vi "Framework Plugin Runtime Test.vi"() -> ()   [LabVIEW 2016]
uses:
  Plugin Runtime.UDP/Plugin Runtime.UDP.lvclass
  Plugin/Plugin.lvclass
  Framework/Framework.lvclass
  <vilib>/platform/TimedLoop/XDataNode/XDataNode.xnode
  <vilib>/Platform/TimedLoop/XDataNode/nitl_modes.ctl
  <vilib>/Platform/TimedLoop/XDataNode/XDNodeRunTimeDep.lvlib
  <vilib>/Platform/TimedLoop/XDataNode/wakeup.ctl
  <vilib>/Platform/TimedLoop/XDataNode/timing_clust.ctl
  Simulated VeriStand Engine/Simulated VeriStand Engine.lvclass
  Typdefs/Decimation Factors.ctl
  <vilib>/NI Veristand/VeriStand Data/Typedefs/Typedefs.Data Types.ctl
  <vilib>/NI Veristand/VeriStand Data/VeriStand Data.lvlib
  <vilib>/NI Veristand/VeriStand Data/Byte Buffer/Byte Buffer.Mapping.ctl
  <vilib>/NI Veristand/VeriStand Data/Byte Buffer/Byte Buffer.lvclass
  Typdefs/Buffer Configuration.ctl
  C:/Git/SourceTree/VeriStand-Data-Sharing-Framework/Prototyping/Plugin Runtime/Plugin Runtime.lvclass
  <vilib>/NI Veristand/Custom Device API/Data Reference.ctl
  <vilib>/NI VeriStand/Custom Device API/Custom Device API.lvlib
panel:
  out "Plugin Base Pointer":u64 format="%016x"
  in  "Engine Loop Rate (Hz)":dbl=100.0 format="%#_13g"
  in  "Engine Channel Count":i64=1000
  in  "Channels per Section":i32=100
  in  "Number of Sections":i32=5
  in  "Plugin Data Offset":T1 format="%.0x"
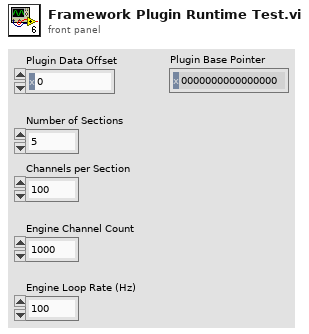
[diagram p1: front panel]
types:
  T1 = typedef "Custom Device API.lvlib/Data Reference.ctl" = i32
  T2 = typedef "Buffer Configuration.ctl" = cluster{"channel mappings":T3[], "rate decimation factors":T5}
  T3 = typedef "VeriStand Data.lvlib/Byte Buffer.lvclass/Byte Buffer.Mapping.ctl" = cluster{"pointer":u64, "count":i64, "buffer offset":u64, "data type":T4}
  T4 = typedef "VeriStand Data.lvlib/Typedefs.Data Types.ctl" = enum16{"Boolean", "Single", "Double", "I8", "I16", "I32", "I64", "U8", "U16", "U32", "U64"}
  T5 = typedef "Decimation Factors.ctl" = cluster{"decimation":u16, "offset":u16}
  T6 = typedef "XDNodeRunTimeDep.lvlib/timing_clust.ctl" = cluster{"Expected End [f-1]":u64, "Actual End [f-1]":u64, "Finished Late? [f-1]":bool, "Expected End [i-1]":u64, "Actual End [i-1]":u64, "Finished Late? [i-1]":bool, "Expected Start [i]":u64, "Actual Start [i]":u64, "Expected Start [f]":u64, "Actual Start [f]":u64, "Source Name":string, "Structure Name":string, "Period":i64, "Deadline":i64, "Offset":i64, "Start":i64, "Priority":i32, "Timeout":i32, "Mode":T7, "Wakeup Reason":T8, "Error":errorcluster, "Source Type":string, "Secondary Source Type":string, "Global End Time":u64, "Global Start Time":u64, "Frame Duration":u64, "Iteration Duration":u64, "Assigned CPU":i32, "I/O Scan Engine Mode":u32}
  T7 = typedef "XDNodeRunTimeDep.lvlib/nitl_modes.ctl" = enum32{"No Change", "Process missed periods, maintain original phase", "Discard missed periods, maintain original phase", "Process missed periods, ignore original phase", "Discard missed periods, ignore original phase"}
  T8 = typedef "XDNodeRunTimeDep.lvlib/wakeup.ctl" = enum32{"Normal", "Aborted", "Asynchronous wakeup", "Timing source error", "Timed loop error", "Timeout"}
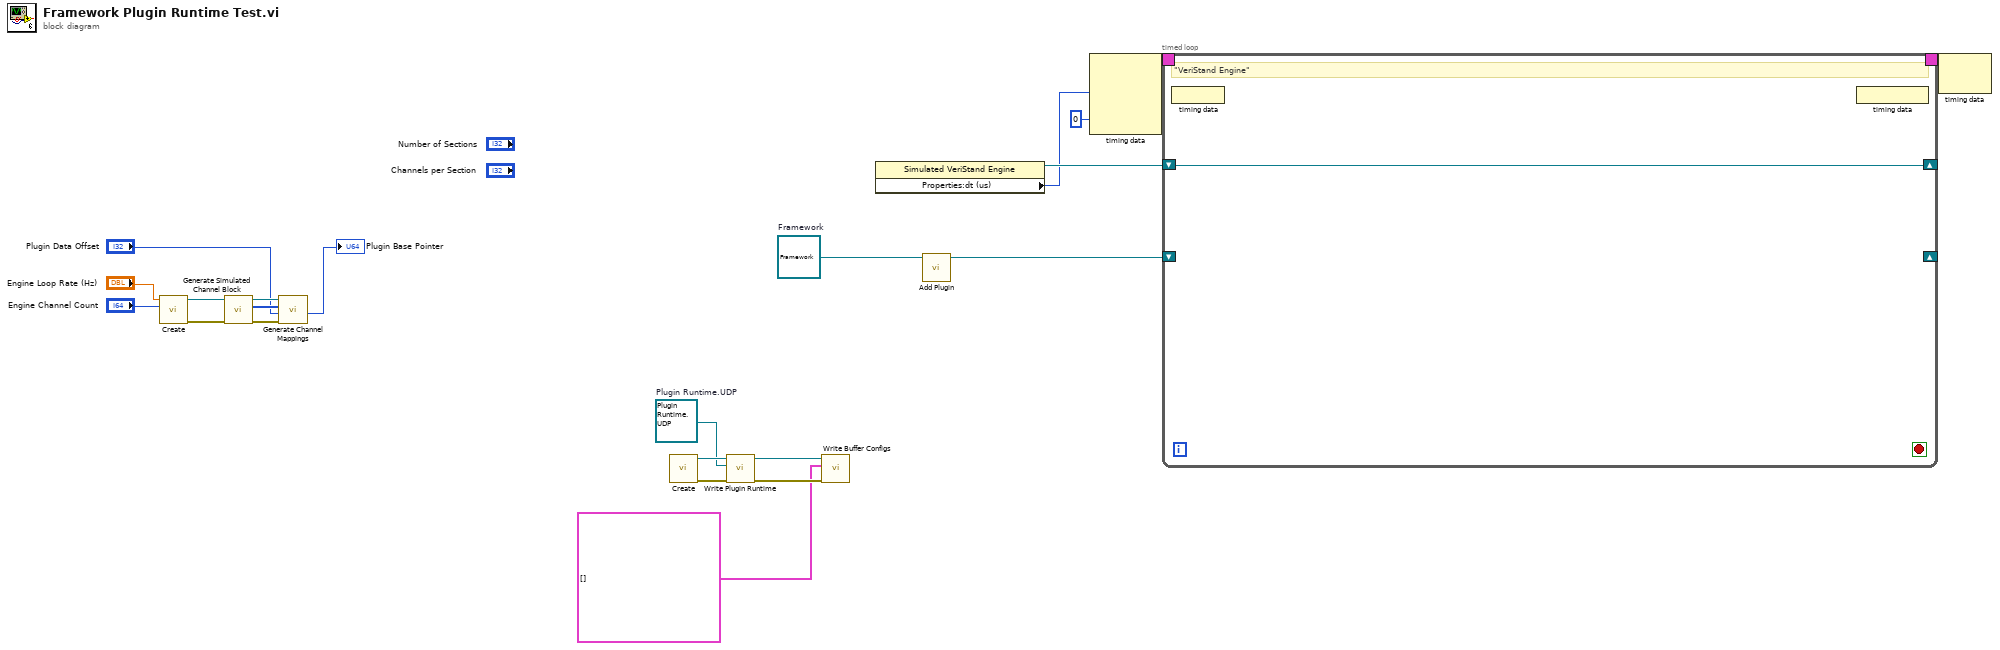
[diagram p0: block diagram]
diagram:
  w12 = refnum<class "Framework.lvclass"> refnum  # Framework
  w13 = refnum<class "Plugin Runtime.UDP.lvclass"> refnum  # Plugin Runtime.UDP
  n1 = call "Create.vi"("Channel Count"="Engine Channel Count", "Loop Rate (Hz)"="Engine Loop Rate (Hz)") -> ("error out"=w6:errorcluster, "Simulated VeriStand Engine out"=w3:refnum<class "Simulated VeriStand Engine.lvclass">)  [unwired: 8 in]
  n2 = call "Generate Simulated Channel Block.vi"("error in (no error)"=w6, "Simulated VeriStand Engine in"=w3) -> ("error out"=w5:errorcluster, "Channels"=w2:T4[], "Simulated VeriStand Engine out"=w4:refnum<class "Simulated VeriStand Engine.lvclass">)  [unwired: 6 in, 1 out]
  n3 = call "Generate Channel Mappings.vi"("error in (no error)"=w5, "Plugin Data Offset"="Plugin Data Offset", "Channels"=w2, "Simulated VeriStand Engine in"=w4) -> ("Base Pointer"=→"Plugin Base Pointer":u64)  [unwired: 4 in, 3 out]
  n4 = call "Create.vi"() -> ("error out"=w14:errorcluster, "Plugin out"=w15:refnum<class "Plugin.lvclass">)  [unwired: 10 in]
  n5 = call "Write Plugin Runtime.vi"("error in (no error)"=w14, "Data Sharing Plugin Runtime"=w13, "Data Sharing Plugin in"=w15) -> ("error out"=w9:errorcluster, "Data Sharing Plugin out"=w10:refnum<class "Plugin.lvclass">)  [unwired: 7 in]
  n6 = call "Write Buffer Configs.vi"("error in (no error)"=w9, "Buffer Configs"=T2[] [], "Plugin in"=w10) -> ()  [unwired: 7 in, 2 out]
  n7 = property class="Simulated VeriStand Engine"() -> (reference out=w18:refnum<class "Simulated VeriStand Engine.lvclass">, "Properties:dt (us)"=w16:i64)  [unwired: 2 in, 1 out]
  n8 = call-dynamic "Add Plugin.vi"("Framework in"=w12) -> ("Framework out"=w11:refnum<class "Framework.lvclass">)  [unwired: 9 in, 1 out]
  n9 = node-c288(w16, 0 ("Processor")) -> (w22:T6)  [unwired: 2 in]
  n10 = timed-loop {
    timing: w22 -> [_]
    timing-out: [_] -> w21
    shift-right: [w23] -> _
    shift-left: w18 -> [w23]
    shift-right: _ -> [_]
    shift-left: w11 -> [_]
    stop <- _ stop-if-true
    # "\"VeriStand Engine\""
    n11 = node-c288() -> ()  [unwired: 1 in]
    n12 = node-c288() -> ()  [unwired: 1 out]
  }
  n13 = node-c288(w21) -> ()  [unwired: 1 out]
